vi "Done.vi"(8 "error in (no error)":errorcluster, 11 "String Control Sink in":refnum<class "String Control Sink.lvclass">) -> (0 "error out":errorcluster)   [LabVIEW 2017, in "String Control Sink.lvclass"]
doc: "--\nCopyright © 2017 Composed SystemsI All rights reserved.\n\nAuthor: Jon McBee <jon.mcbee@composed.io>\n\nThis library is provided \"AS IS\" ,WITHOUT WARRANTIES OR\nCONDITIONS OF ANY KIND, either express or implied.\n\nComposed Systems -- composed.io\n\nStream 0.0.1.1\nJon McBee - Composed Systems\nCopyright (c) 2017, Composed Systems"
uses:
  <vilib>/gpm_packages/@cs/event-logger/Source/String Control Sink/String Control Sink.lvclass
  <vilib>/gpm_packages/@cs/event-logger/Source/String Control Sink/String Control Sink.lvclass/String Control Sink.ctl
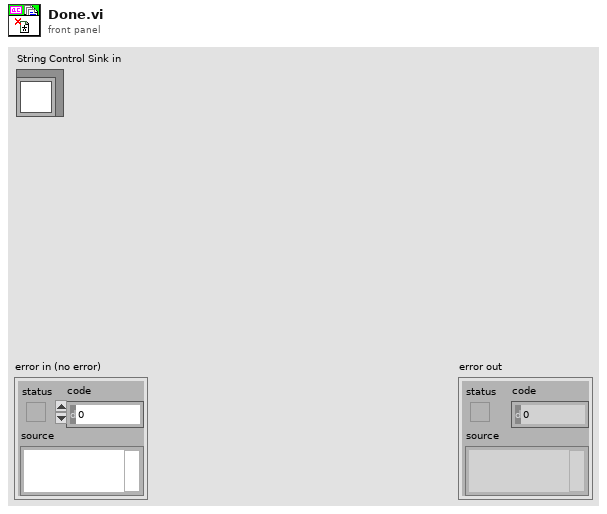
[diagram p1: front panel]
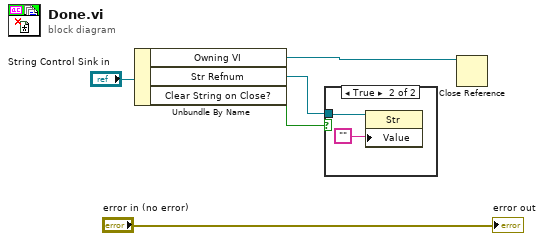
[diagram p0: block diagram]
diagram:
  n1 = Unbundle By Name("String Control Sink in") -> ("Owning VI"=w3:refnum<vi>, "Str Refnum"=w1:refnum<vi>, "Clear String on Close?"=w2:bool)
  n2 = case shown="True" w2 {
    tunnel: w1 -> [_ w7]
    frame False {
    }
    frame True {
      n3 = property class="Str"(reference=w7, "Value"="") -> ()  [unwired: 1 in, 2 out]
    }
  }
  n4 = Close Reference(reference=w3) -> ()  [unwired: 1 in, 1 out]
  "error out" <- "error in (no error)"
